vi "T7MOD_Write_UINT16_Registers.vi"(7 "UINT16 to Write":u16[](array[numeric]), 8 "error in":errorcluster, 9 "Starting Address":i32=55110, 10 "Remote Port":u16=502, 11 "Remote IP Address":string="192.168.1.15") -> (0 "error out":errorcluster, 1 "Written At":timestamp)   [LabVIEW 2018]
panel:
  # "Input"
  # "TCP Parameters"
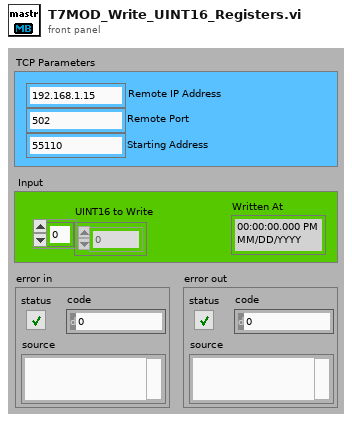
[diagram p1: front panel]
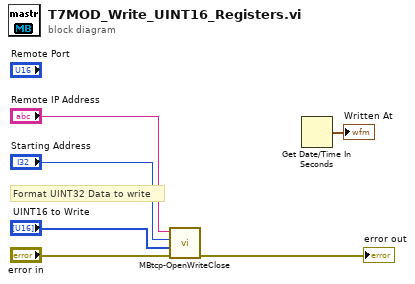
[diagram p0: block diagram]
diagram:
  # "Format UINT32 Data to write"
  n1 = call "MBtcp-OpenWriteClose.vi"("error in (no error)"="error in", "Values"="UINT16 to Write", "RegisterAddr"="Starting Address", "IP Address(:port)"="Remote IP Address") -> ("error out"=→"error out":errorcluster)  [unwired: 7 in]
  n2 = Get Date/Time In Seconds() -> (seconds since 1Jan1904=→"Written At":timestamp)
